vi "Day 15 - Part two.vi"() -> ()   [LabVIEW 2023]
panel:
  out "Tuning frequency":u64
  in  "test":bool
  in  "test input":string="Sensor at x=2, y=18: closest beacon is at x=-2, y=15\nSensor at x=9, y=16: closest beacon is at x=10, y=16\nSensor at x=13, y=2: closest beacon is at x=15, y=3\nSensor at x=12, y=14: closest beacon is at x=10, y=16\nSensor at x=10, y=20: closest beacon is at x=10, y=16\nSensor at x=14, y=17: closest beacon is at x=10, y=16\nSensor at x=8, y=7: closest beacon is at x=2, y=10\nSensor at x=2, y=0: closest beacon is at x=2, y=10\nSensor at x=0, y=11: closest beacon is at x=2, y=10\nSensor at x=20, y=14: closest beacon is at x=25, y=17\nSensor at x=17, y=20: closest beacon is at x=21, y=22\nSensor at x=16, y=7: closest beacon is at x=15, y=3\nSensor at x=14, y=3: closest beacon is at x=15, y=3\nSensor at x=20, y=1: closest beacon is at x=15, y=3"
  in  "input":string="Sensor at x=3289936, y=2240812: closest beacon is at x=3232809, y=2000000\nSensor at x=30408, y=622853: closest beacon is at x=-669401, y=844810\nSensor at x=3983196, y=3966332: closest beacon is at x=3232807, y=4625568\nSensor at x=929672, y=476353: closest beacon is at x=-669401, y=844810\nSensor at x=1485689, y=3597734: closest beacon is at x=1951675, y=3073734\nSensor at x=69493, y=1886070: closest beacon is at x=-669401, y=844810\nSensor at x=2146060, y=3999371: closest beacon is at x=2300657, y=4128792\nSensor at x=3228558, y=3890086: closest beacon is at x=3232807, y=4625568\nSensor at x=3031444, y=2295853: closest beacon is at x=2928827, y=2611422\nSensor at x=374444, y=3977240: closest beacon is at x=-888612, y=4039783\nSensor at x=1207660, y=2710720: closest beacon is at x=1951675, y=3073734\nSensor at x=3851310, y=61626: closest beacon is at x=4807592, y=976495\nSensor at x=3195193, y=3022787: closest beacon is at x=2928827, y=2611422\nSensor at x=1784895, y=2111901: closest beacon is at x=1951675, y=3073734\nSensor at x=2894075, y=2427030: closest beacon is at x=2928827, y=2611422\nSensor at x=3301867, y=803327: closest beacon is at x=3232809, y=2000000\nSensor at x=2506616, y=3673347: closest beacon is at x=2300657, y=4128792\nSensor at x=2628426, y=3054377: closest beacon is at x=1951675, y=3073734\nSensor at x=2521975, y=1407505: closest beacon is at x=3232809, y=2000000\nSensor at x=2825447, y=2045173: closest beacon is at x=3232809, y=2000000\nSensor at x=2261212, y=2535886: closest beacon is at x=2928827, y=2611422\nSensor at x=3956000, y=1616443: closest beacon is at x=3232809, y=2000000\nSensor at x=3870784, y=2872668: closest beacon is at x=2928827, y=2611422\n"
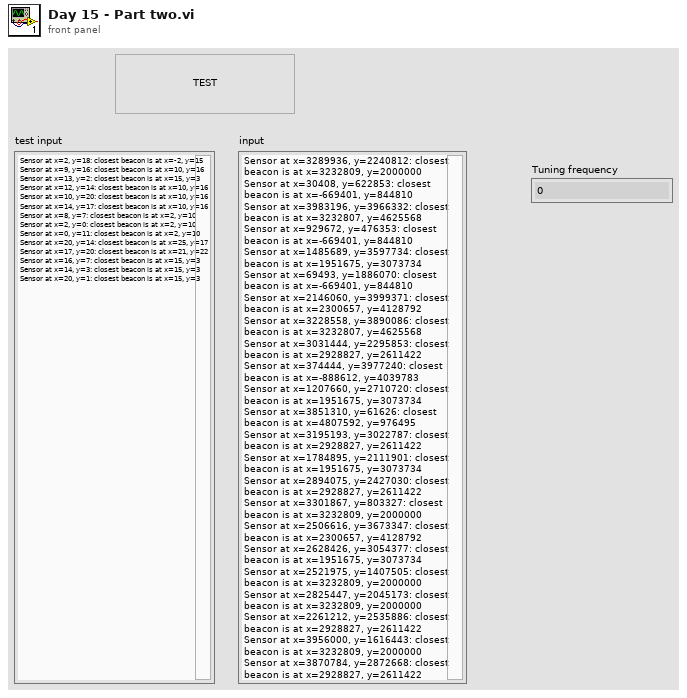
[diagram p1: front panel]
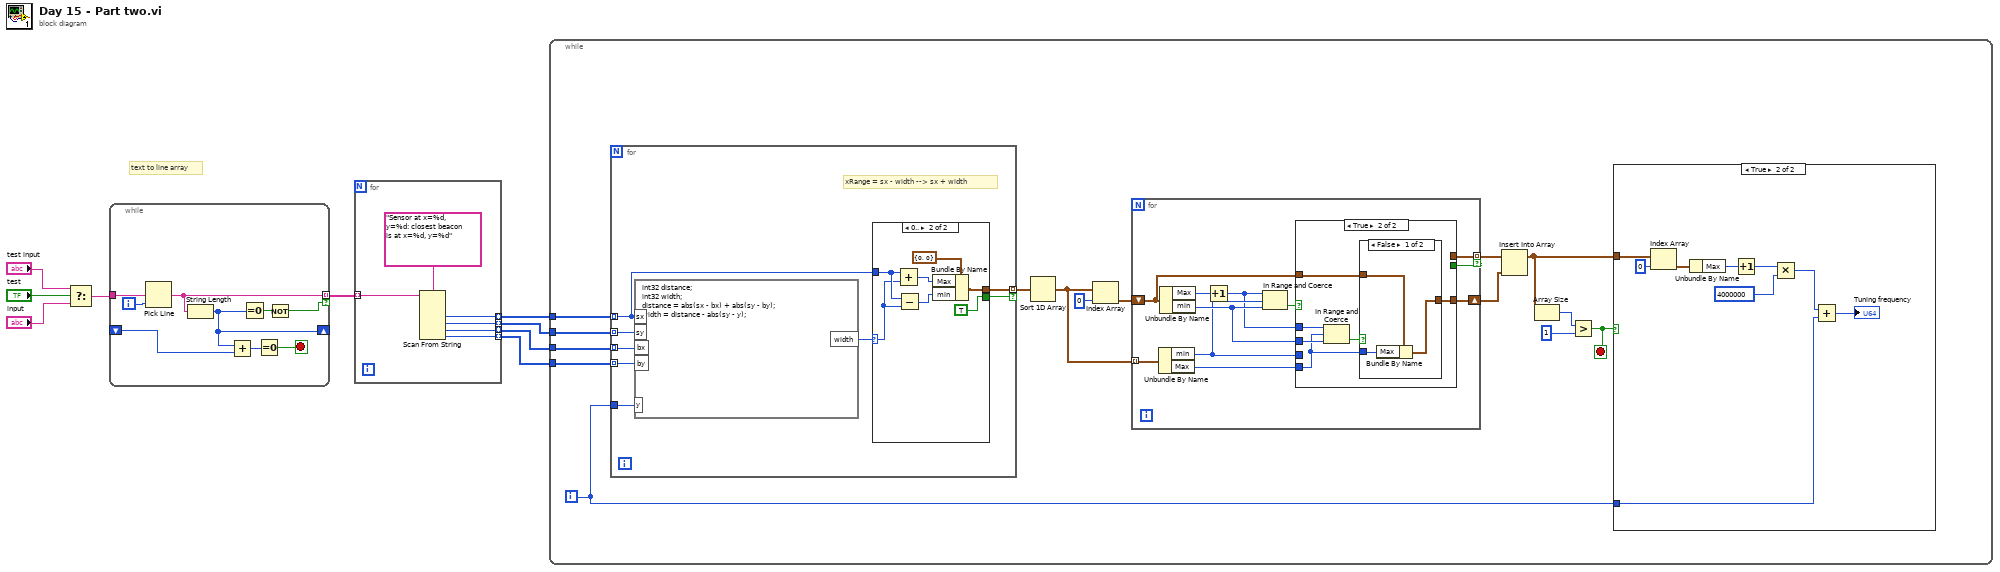
[diagram p0: block diagram]
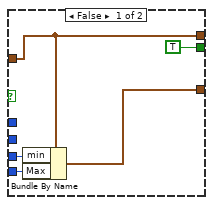
[diagram p3: hidden frame]
diagram:
  # "text to line array"
  n1 = Select(t="test input", s="test", f="input") -> (s? t:f=w7:string)
  n2 = while {
    tunnel: w7 -> [w17]
    tunnel: [w10] -> w5 mode=indexing if=w16
    shift-right: [w13] -> _
    shift-left: _ -> [w14]
    i -> [w18]
    stop <- w11 stop-if-true
    n3 = Pick Line(multi-line string=w17, line index=w18) -> (output string=w10:string)  [unwired: 1 in]
    n4 = String Length(string=w10) -> (length=w13:i32)
    n5 = Add(x=w13, y=w14) -> (x+y=w15:i32)
    n6 = Equal To 0?(x=w13) -> (x = 0?=w12:bool)
    n7 = Equal To 0?(x=w15) -> (x = 0?=w11:bool)
    n8 = Not(x=w12) -> (.not. x?=w16:bool)
  }
  n9 = for {
    tunnel: w5 -> [w24] mode=indexing
    tunnel: [w23] -> w1 mode=indexing
    tunnel: [w22] -> w2 mode=indexing
    tunnel: [w21] -> w3 mode=indexing
    tunnel: [w20] -> w4 mode=indexing
    n10 = Scan From String(format string="Sensor at x=%d, y=%d: closest beacon is at x=%d, y=%d", input string=w24) -> (output 1=w23:i32, output 2=w22:i32, output 3=w21:i32, output 4=w20:i32)  [unwired: 6 in, 3 out]
  }
  n11 = while {
    tunnel: w4 -> [w31]
    tunnel: w3 -> [w30]
    tunnel: w2 -> [w29]
    tunnel: w1 -> [w28]
    i -> [w26]
    stop <- w25 stop-if-true
    n12 = for {
      tunnel: w26 -> [w47]
      tunnel: [w45] -> w39 mode=indexing if=w44
      tunnel: w31 -> [w43] mode=indexing
      tunnel: w30 -> [w42] mode=indexing
      tunnel: w29 -> [w41] mode=indexing
      tunnel: w28 -> [w40] mode=indexing
      # "xRange = sx - width --> sx + width"
      n13 = formula code="int32 distance;\nint32 width;\ndistance = abs(sx - bx) + abs(sy - by);\nwidth = distance - abs(sy - y);"("sx"=w40, "sy"=w41, "bx"=w42, "by"=w43, "y"=w47) -> ("width"=w46:i32)
      n14 = case shown="0.." w46 {
        selector: w46 -> [_ w53]
        tunnel: w40 -> [_ w54]
        tunnel: [_ w52] -> w45
        tunnel: [_ TRUE] -> w44
        frame -1, Default {
        }
        frame 0.. {
          n15 = Add(x=w54, y=w53) -> (x+y=w49:i32)
          n16 = Subtract(x=w54, y=w53) -> (x-y=w50:i32)
          n17 = Bundle By Name(cluster=cluster{"min":i32, "Max":i32} {"min"=0, "Max"=0} ("output cluster"), "Max"=w49, "min"=w50) -> (w52:cluster{"min":i32, "Max":i32})
        }
      }
    }
    n18 = Sort 1D Array(array=w39) -> (sorted array=w36:cluster{"min":i32, "Max":i32}[])
    n19 = Index Array(array=w36, index=0) -> (element=w35:cluster{"min":i32, "Max":i32})
    n20 = for {
      tunnel: w36 -> [w64] mode=indexing
      shift-right: [w59] -> w37
      shift-left: w35 -> [w60]
      tunnel: [w58] -> w38 mode=indexing if=w57
      n21 = Unbundle By Name(w64) -> ("min"=w56:i32, "Max"=w61:i32)
      n22 = Unbundle By Name(w60) -> ("Max"=w62:i32, "min"=w63:i32)
      n23 = Increment(x=w62) -> (x+1=w55:i32)
      n24 = In Range and Coerce(upper limit=w55, x=w56, lower limit=w63) -> (In Range?=w65:bool)  [unwired: 1 out]
      n25 = case shown="True" w65 {
        tunnel: w63 -> [_ w74]
        tunnel: w55 -> [_ w76]
        tunnel: w61 -> [w69 w72]
        tunnel: w60 -> [w66 w73]
        tunnel: [w67 w71] -> w59
        tunnel: [w66 _] -> w58
        tunnel: [TRUE _] -> w57
        tunnel: w56 -> [w68 _]
        frame False {
          n26 = Bundle By Name(cluster=w66, "min"=w68, "Max"=w69) -> (w67:cluster{"min":i32, "Max":i32})
        }
        frame True {
          n27 = In Range and Coerce(upper limit=w76, x=w72, lower limit=w74) -> (In Range?=w75:bool)  [unwired: 1 out]
          n28 = case shown="False" w75 {
            tunnel: w73 -> [w79 w80]
            tunnel: w72 -> [w78 _]
            tunnel: [w77 w80] -> w71
            frame False {
              n29 = Bundle By Name(cluster=w79, "Max"=w78) -> (w77:cluster{"min":i32, "Max":i32})
            }
            frame True {
            }
          }
        }
      }
    }
    n30 = Insert Into Array(array=w38, new element=w37) -> (w27:cluster{"min":i32, "Max":i32}[])  [unwired: 1 in]
    n31 = Array Size(array=w27) -> (size(s)=w33:i32)
    n32 = Greater?(x=w33, y=1) -> (0:w25:bool)
    n33 = case shown="True" w25 {
      tunnel: w27 -> [_ w83]
      tunnel: w26 -> [_ w81]
      frame False {
      }
      frame True {
        n34 = Index Array(array=w83, index=0) -> (element=w88:cluster{"min":i32, "Max":i32})
        n35 = Unbundle By Name(w88) -> ("Max"=w82:i32)
        n36 = Increment(x=w82) -> (x+1=w87:i32)
        n37 = Multiply(x=w87, y=u64 4000000) -> (x*y=w86:u64)
        n38 = Add(x=w86, y=w81) -> (x+y=→"Tuning frequency":u64)
      }
    }
  }
